vi "niRFUtil WFM Aggregate Waveforms.vi"   [LabVIEW 2015, in "niRFUtil.lvlib"]
doc: "(c) Copyright 2006, National Instruments, Inc. This VI may not be duplicated, sold, or distributed without written consent from National Instruments."
uses:
  niRFUtil.lvlib
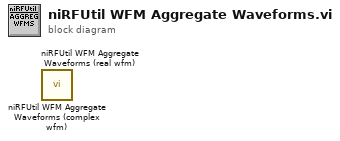
[diagram p0: block diagram]
diagram:
  n1 = call "niRFUtil WFM Aggregate Waveforms (complex wfm).vi"() -> ()  [unwired: 4 in, 1 out]
  n2 = call "niRFUtil WFM Aggregate Waveforms (real wfm).vi"() -> ()  [unwired: 4 in, 1 out]
